vi "Simple Camera Test.vi"() -> ()   [LabVIEW 2017]
uses:
  <vilib>/userdefined/High Color/IMAQdx.ctl
  <vilib>/vision/driver/NI_Vision_Acquisition_Software.lvlib
panel:
  out "Image":T1(plugin-control)
  out "Camera Information Array":T2(array[cluster]) {"BusType" format="%x"; "SerialNumberLow" format="%.0x"; "SerialNumberHigh" format="%.0x"}
  out "error out":errorcluster
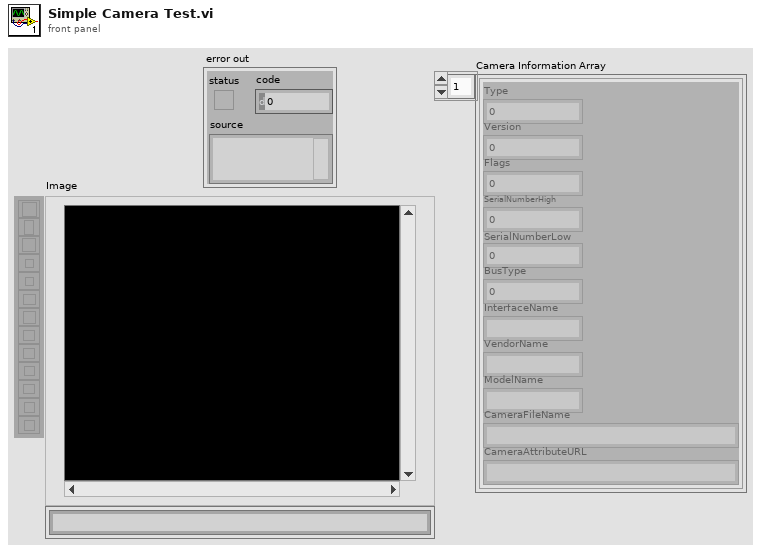
[diagram p1: front panel]
types:
  T1 = typedef "IMAQ Image.ctl" = refnum<image>
  T2 = cluster{"Type":u32, "Version":u32, "Flags":u32, "SerialNumberHigh":u32, "SerialNumberLow":u32, "BusType":u32, "InterfaceName":string, "VendorName":string, "ModelName":string, "CameraFileName":string, "CameraAttributeURL":string}[]
  T3 = typedef "IMAQdx.ctl" = refnum<k21>
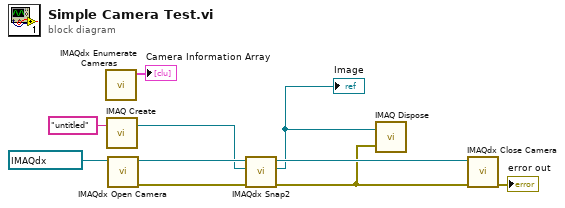
[diagram p0: block diagram]
diagram:
  n1 = call <vilib>:"IMAQdx Enumerate Cameras.vi"() -> ("Camera Information Array"=→"Camera Information Array":T2)  [unwired: 10 in, 1 out]
  n2 = call "IMAQ Create"("Image Name"="untitled") -> ("New Image"=w2:T1)  [unwired: 4 in, 1 out]
  n3 = call <vilib>:"IMAQdx Open Camera.vi"("Session In"=T3 "cam0 (3)") -> ("error out"=w3:errorcluster, "Session Out"=w6:T3)  [unwired: 9 in]
  n4 = call <vilib>:"IMAQdx Snap2.vi"("error in"=w3, "Image In"=w2, "Session In"=w6) -> ("error out"=w4:errorcluster, "Image Out"=w1:T1, "Session Out"=w5:T3)  [unwired: 6 in]
  "Image" <- w1
  n5 = call "IMAQ Dispose"("Image"=w1, "error in (no error)"=w4) -> ()  [unwired: 4 in, 1 out]
  n6 = call <vilib>:"IMAQdx Close Camera.vi"("error in"=w4, "Session In"=w5) -> ("error out"=→"error out":errorcluster)  [unwired: 9 in]
